vi "Read.vi"(8 "error in (no error)":errorcluster, 9 "Sample Rate [Hz]":dbl=1000.0 min=1000.0 max=30000.0, 10 "Number of Samples":u32=1000, 11 "AudioIn (N Samples) Ref In":T1) -> (0 "error out":errorcluster, 2 "Values":dbl[][](array[numeric]), 3 "AudioIn (N Samples) Ref Out":T1)   [LabVIEW 2021, in "AudioIn Block.lvlib"]
doc: "Reads values from one or more audio input channels. Use this VI to read multiple samples for each channel at one time."
uses:
  <vilib>/myRIO/Instrument Drivers/Onboard IO/AudioIn Block/AudioIn Block.lvlib
  <vilib>/myRIO/Instrument Drivers/Onboard IO/AudioIn Block/typedefs/AudioIn Block Reference.ctl
  <vilib>/myRIO/Common/Instrument Driver Framework/Utilities/typedefs/myRIO Generic Hardware Reference.ctl
  <vilib>/myRIO/Common/Instrument Driver Framework/Utilities/typedefs/Hardware Version Enum.ctl
  <vilib>/myRIO/Common/Instrument Driver Framework/Utilities/typedefs/myRIO v1.0 Reference.ctl
  <vilib>/myRIO/Common/Instrument Driver Framework/Utilities/typedefs/Generic FPGA Reference.ctl
  <vilib>/myRIO/Common/Instrument Driver Framework/myRIO v1.0/AudioIn Block/typedefs/AudioIn Block Channels List.ctl
  <vilib>/myRIO/Common/Instrument Driver Framework/myRIO v1.0/AudioIn Block/typedefs/AudioIn Block Channels Enum.ctl
  <vilib>/myRIO/Common/Instrument Driver Framework/Utilities/typedefs/Analog Scaling Constants.ctl
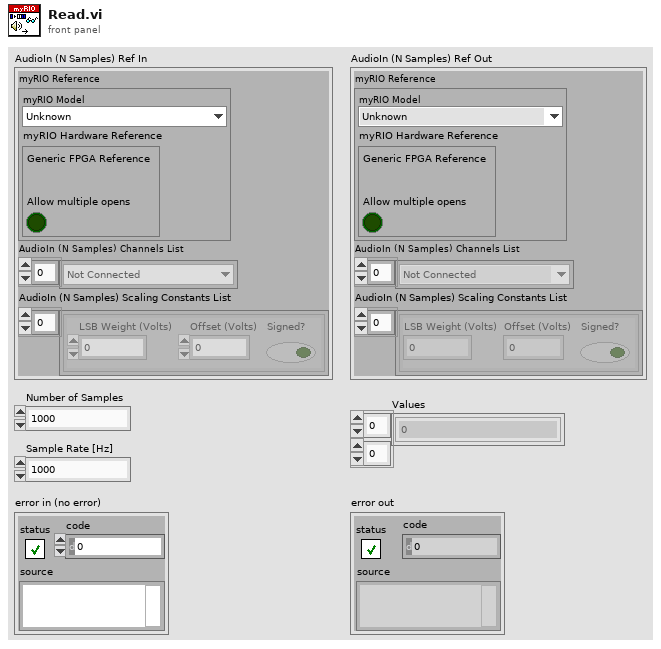
[diagram p1: front panel]
types:
  T1 = typedef "AudioIn Block.lvlib/AudioIn Block Reference.ctl" = cluster{"myRIO Reference":T2, "AudioIn (N Samples) Channels List":T6, "AudioIn (N Samples) Scaling Constants List":T8[]}
  T2 = typedef "myRIO Generic Hardware Reference.ctl" = cluster{"myRIO Model":T3, "myRIO Hardware Reference":T4}
  T3 = typedef "Hardware Version Enum.ctl" = enum16{"Unknown", "myRIO-1900", "myRIO-1950", "roboRIO", "NI ELVIS RIO CM", "ELVIS III"}
  T4 = typedef "myRIO v1.0 Reference.ctl" = cluster{"Generic FPGA Reference":T5, "Allow multiple opens":bool}
  T5 = typedef "Generic FPGA Reference.ctl" = refnum<k20>
  T6 = typedef "AudioIn Block Channels List.ctl" = T7[]
  T7 = typedef "AudioIn Block Channels Enum.ctl" = enum16{"Not Connected", "AudioIn/Left (N Samples)", "AudioIn/Right (N Samples)"}
  T8 = typedef "Analog Scaling Constants.ctl" = cluster{"LSB Weight (Volts)":dbl, "Offset (Volts)":dbl, "Signed?":bool}
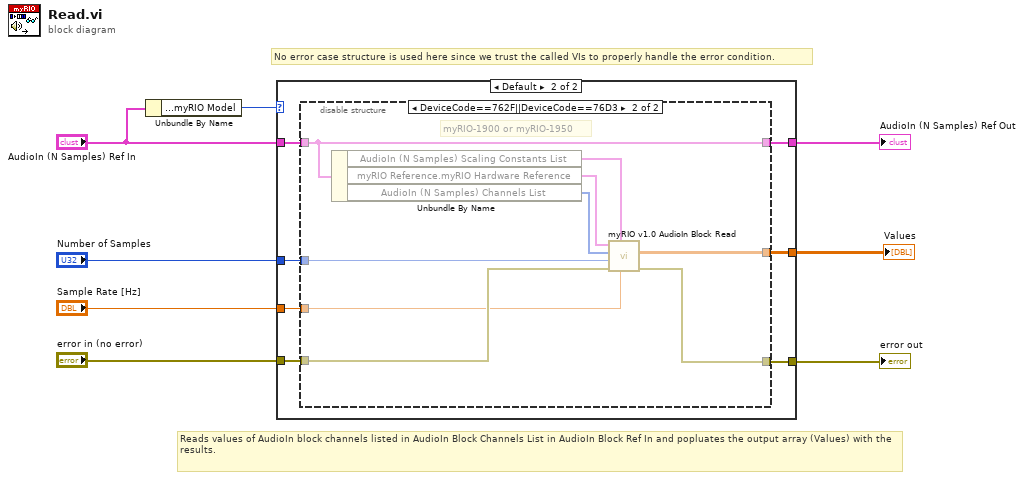
[diagram p0: block diagram]
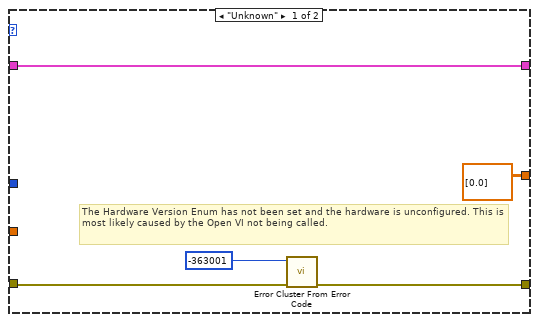
[diagram p2: hidden frame]
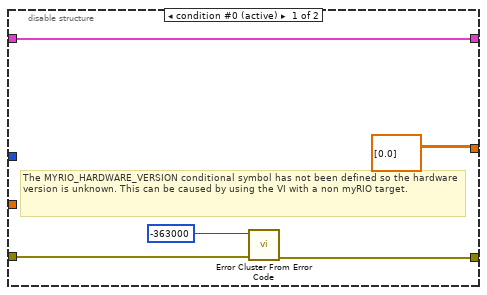
[diagram p3: hidden frame]
diagram:
  # "No error case structure is used here since we trust the called VIs to properly handle the error condition."
  # "Reads values of AudioIn block channels listed in AudioIn Block Channels List in AudioIn Block Ref In and popluates the output array (Values) with the results."
  n1 = Unbundle By Name("AudioIn (N Samples) Ref In") -> ("myRIO Reference.myRIO Model"=w3:T3)
  n2 = case shown="Default" w3 {
    tunnel: [w11 w20] -> w5
    tunnel: "AudioIn (N Samples) Ref In" -> [w10 w19]
    tunnel: "error in (no error)" -> [w12 w18]
    tunnel: [w10 w17] -> w6
    tunnel: [dbl[][] [[0.0]] w16] -> w4
    tunnel: "Sample Rate [Hz]" -> [_ w15]
    tunnel: "Number of Samples" -> [_ w14]
    frame "Unknown" {
      # "The Hardware Version Enum has not been set and the hardware is unconfigured. This is most likely caused by the Open VI not being called."
      n3 = call <vilib>:"Error Cluster From Error Code.vi"("error in (no error)"=w12, "error code (0)"=-363001) -> ("error out"=w11:errorcluster)  [unwired: 7 in]
    }
    frame Default {
      n4 = disable-structure shown="DeviceCode==762F||DeviceCode==76D3" {
        disable-tunnel: w19 -> [w22 w27]
        disable-tunnel: [w25 w33] -> w20
        disable-tunnel: w18 -> [w23 w34]
        disable-tunnel: [w22 w27] -> w17
        disable-tunnel: [dbl[][] [[0.0]] ("dbl Scaled Value List") w31] -> w16
        disable-tunnel: w15 -> [_ w28]
        disable-tunnel: w14 -> [_ w29]
        frame condition #0 (active) {
          # "The MYRIO_HARDWARE_VERSION conditional symbol has not been defined so the hardware version is unknown. This can be caused by using the VI with a non myRIO target."
          n5 = call <vilib>:"Error Cluster From Error Code.vi"("error in (no error)"=w23, "error code (0)"=-363000) -> ("error out"=w25:errorcluster)  [unwired: 7 in]
        }
        frame condition #1 {
          # "myRIO-1900 or myRIO-1950"
          n6 = Unbundle By Name(w27) -> ("AudioIn (N Samples) Scaling Constants List"=w26:T8[], "myRIO Reference.myRIO Hardware Reference"=w32:T4, "AudioIn (N Samples) Channels List"=w30:T6)
          n7 = call <vilib>:"myRIO v1.0 AudioIn Block Read.vi"("AudioIn FIFO Sample Rate"=w28, "Scale Constants Array"=w26, "error in (no error)"=w34, "Number of Samples"=w29, "AudioIn (N Samples) Channel List"=w30, "myRIO Ref In"=w32) -> ("error out"=w33:errorcluster, "dbl Scaled Value List"=w31:dbl[][])  [unwired: 3 in, 1 out]
        }
      }
    }
  }
  "AudioIn (N Samples) Ref Out" <- w6
  "error out" <- w5
  "Values" <- w4
